vi "Waveform Peak Detection for N Chan.vi"(4 "end of data (T)":bool=TRUE, 6 "initialize (T)":bool=TRUE, 7 "peaks/valleys":u16(ring) items=["Peaks", "Valleys"], 8 "error in":errorcluster, 9 "width":i32=3 min=3, 10 "threshold":dbl format="%.2p", 11 "Signals In":waveform(dbl)[](array[waveform])) -> (0 "error out":errorcluster, 1 "2nd Derivatives":cluster{"2nd Derivatives":dbl[]}[](array[cluster]) {"2nd Derivatives" format="%.2p"}, 2 "Amplitudes":cluster{"Amplitudes":dbl[]}[](array[cluster]) {"Amplitudes" format="%.2p"}, 3 "Locations":cluster{"Locations":dbl[]}[](array[cluster]) {"Locations" format="%.2p"}, 5 "# found":i32[](array[numeric]))   [LabVIEW 2020, in "NI_MAPro.lvlib"]
doc: "Finds the locations, amplitudes, and second derivatives of peaks and valleys in <B>Signal In</B>. Wire data to the <B>Signal In</B> input to determine the polymorphic instance to use or manually select the instance."
uses:
  NI_MAPro.lvlib
  NI_MABase.lvlib
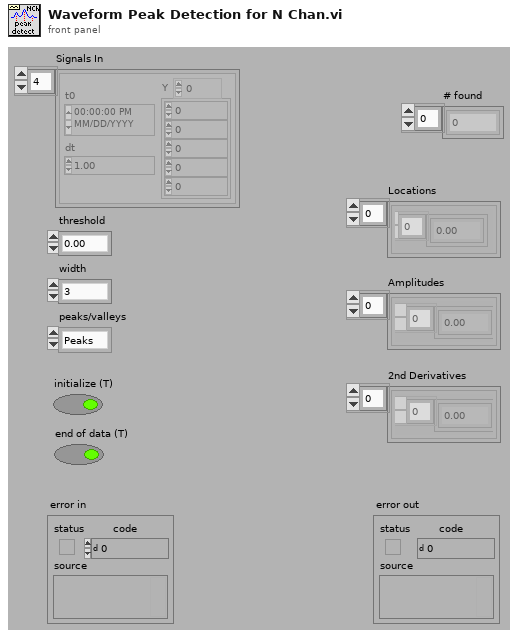
[diagram p1: front panel]
types:
  T1 = cluster{"PEAKINT":cluster{"Span":i32, "Index":i32, "NHistoryPts":i32, "Len":i32, "PrevSign":i32, "unused":i32, "RinvQt (pointer)":u32, "FitBuffer (pointer)":u32, "History (pointer)":u32, "PrevCoeff (pointer)":u32, "Data (pointer)":u32, "slack for RinvQt":u32, "slack for FitBuffer":u32, "slack for History":u32, "slack for PrevCoeff":u32, "slack for Data":u32}, "SavedData":dbl[]}
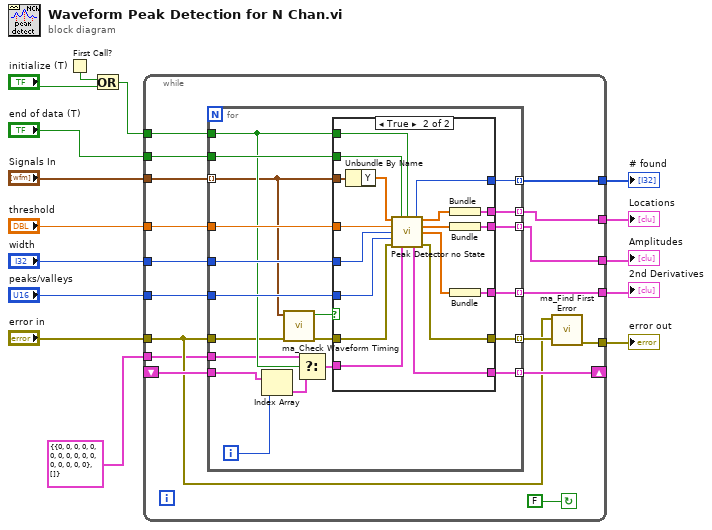
[diagram p0: block diagram]
diagram:
  n1 = First Call?() -> (First Call?: T/F=w9:bool)
  n2 = Or(x=w9, y="initialize (T)") -> (x .or. y?=w8:bool)
  n3 = while {
    tunnel: "error in" -> [w18]
    tunnel: "threshold" -> [w32]
    tunnel: "peaks/valleys" -> [w31]
    tunnel: w8 -> [w30]
    tunnel: "end of data (T)" -> [w29]
    tunnel: [w28] -> w5
    tunnel: [w27] -> w3
    tunnel: [w26] -> w4
    tunnel: [w25] -> w6
    tunnel: "width" -> [w24]
    tunnel: "Signals In" -> [w23]
    shift-right: [w20] -> _
    shift-left: _ -> [w21]
    tunnel: [w17] -> w2
    tunnel: T1 {"PEAKINT"={"Span"=0, "Index"=0, "NHistoryPts"=0, "Len"=0, "PrevSign"=0, "unused"=0, "RinvQt (pointer)"=0, "FitBuffer (pointer)"=0, "History (pointer)"=0, "PrevCoeff (pointer)"=0, "Data (pointer)"=0, "slack for RinvQt"=0, "slack for FitBuffer"=0, "slack for History"=0, "slack for PrevCoeff"=0, "slack for Data"=0}, "SavedData"=[]} ("state info") -> [w16]
    stop <- FALSE continue-if-true
    n4 = for {
      tunnel: w18 -> [w35]
      tunnel: w32 -> [w52]
      tunnel: w31 -> [w51]
      tunnel: w30 -> [w40]
      tunnel: w29 -> [w50]
      tunnel: [w45] -> w28 mode=indexing
      tunnel: [w44] -> w27 mode=indexing
      tunnel: [w43] -> w26 mode=indexing
      tunnel: [w49] -> w25 mode=indexing
      tunnel: w24 -> [w48]
      tunnel: [w47] -> w19 mode=indexing
      tunnel: w23 -> [w34] mode=indexing
      tunnel: w21 -> [w38]
      tunnel: [w46] -> w20 mode=indexing
      tunnel: w16 -> [w39]
      i -> [w42]
      n5 = Index Array(array=w38, index=w42) -> (element=w41:T1)
      n6 = call "ma_Check Waveform Timing.vi"("error in (no error)"=w35, "signal in"=w34) -> ("error out"=w36:errorcluster, "timing ok"=w33:bool)  [unwired: 1 in, 7 out]
      n7 = Select(t=w39, s=w40, f=w41) -> (s? t:f=w37:T1)
      n8 = case shown="True" w33 {
        tunnel: w36 -> [w54 w72]
        tunnel: w52 -> [_ w71]
        tunnel: w51 -> [_ w70]
        tunnel: w50 -> [_ w69]
        tunnel: [_ w65] -> w49
        tunnel: w48 -> [_ w64]
        tunnel: [w54 w63] -> w47
        tunnel: w34 -> [_ w62]
        tunnel: [w53 w60] -> w46
        tunnel: [_ w59] -> w45
        tunnel: [_ w58] -> w44
        tunnel: [_ w57] -> w43
        tunnel: w40 -> [_ w56]
        tunnel: w37 -> [w53 w55]
        frame False {
        }
        frame True {
          n9 = Unbundle By Name(w62) -> ("Y"=w61:dbl[])
          n10 = call "Peak Detector no State.vi"("X"=w61, "end of data (T)"=w69, "initialize (T)"=w56, "threshold"=w71, "width"=w64, "peaks/valleys"=w70, "error in"=w72, "state info"=w55) -> ("# found"=w65:i32, "Locations"=w68:dbl[], "Amplitudes"=w67:dbl[], "2nd Derivatives"=w66:dbl[], "state info"=w60:T1, "error out"=w63:errorcluster)  [unwired: 2 out]
          n11 = Bundle("Locations"=w68) -> (w59:cluster{"Locations":dbl[]})  [unwired: 1 in]
          n12 = Bundle("Amplitudes"=w67) -> (w58:cluster{"Amplitudes":dbl[]})  [unwired: 1 in]
          n13 = Bundle("2nd Derivatives"=w66) -> (w57:cluster{"2nd Derivatives":dbl[]})  [unwired: 1 in]
        }
      }
    }
    n14 = call "ma_Find First Error.vi"("error array in"=w19, "error in 1 (no error)"=w18) -> ("error out"=w17:errorcluster)  [unwired: 2 in, 3 out]
  }
  "error out" <- w2
  "# found" <- w6
  "Locations" <- w5
  "2nd Derivatives" <- w4
  "Amplitudes" <- w3
